vi "DMX.vi"(0 "Port Name":string, 1 "DMX channel no.":u8, 2 "Set value:":u8, 4 "Channel Name":string) -> (5 "Achieved value:":i32, 6 "error":bool)   [LabVIEW 2010]
panel:
  out "Read":string
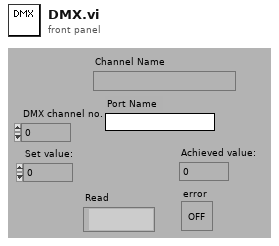
[diagram p1: front panel]
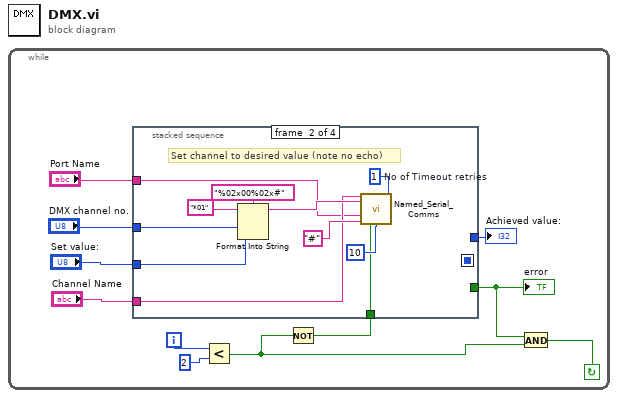
[diagram p0: block diagram]
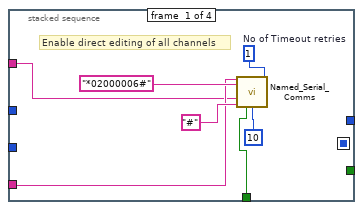
[diagram p2: hidden frame]
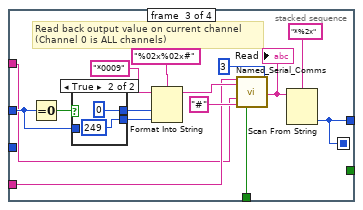
[diagram p3: hidden frame]
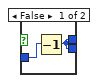
[diagram p4: hidden frame]
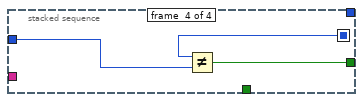
[diagram p5: hidden frame]
diagram:
  n1 = while {
    i -> [w7]
    stop <- w4 continue-if-true
    n2 = Less?(x=w7, y=2) -> (x < y?=w2:bool)
    n3 = Not(x=w2) -> (.not. x?=w1:bool)
    n4 = stacked-sequence {
      seq-local: [_ _ w34 _] -> [_ _ _ w51]
      tunnel: "DMX channel no." -> [_ w25 w37 _]
      tunnel: [_ _ w34 _] -> w10
      tunnel: [_ _ _ w50] -> w5
      tunnel: "Set value:" -> [_ w23 _ w49]
      tunnel: "Channel Name" -> [w15 w22 w33 _]
      tunnel: "Port Name" -> [w13 w20 w31 _]
      tunnel: w1 -> [w12 w19 w30 _]
      frame #0 {
        w14 = 1  # No of Timeout retries
        # "Enable direct editing of all channels"
        n5 = call "Named_Serial_Comms.vi"("Channel Name"=w15, "Write String"="*02000006#", "Timeout/ms"=u32 10, "!Timeout retries"=w14, "Port Name"=w13, "Term Grep"="#" ("Terminator"), "Log Errors?"=w12) -> ()  [unwired: 2 in, 7 out]
      }
      frame #1 {
        w21 = 1  # No of Timeout retries
        # "Set channel to desired value (note no echo)"
        n6 = Format Into String(format string="%02x00%02x#", initial string="*01", w25, w23) -> (resulting string=w27:string)  [unwired: 1 in, 1 out]
        n7 = call "Named_Serial_Comms.vi"("Channel Name"=w22, "Write String"=w27, "Timeout/ms"=u32 10, "!Timeout retries"=w21, "Port Name"=w20, "Term Grep"="#" ("Terminator"), "Log Errors?"=w19) -> ()  [unwired: 2 in, 7 out]
      }
      frame #2 {
        # "Read back output value on current channel\n(Channel 0 is ALL channels)"
        n8 = Equal To 0?(x=w37) -> (x = 0?=w38:bool)
        n9 = case shown="True" w38 {
          tunnel: w37 -> [w46 _]
          tunnel: [w45 u8 0 ("t")] -> w36
          tunnel: [w45 u8 249] -> w35
          frame False {
            n10 = Decrement(x=w46) -> (x-1=w45:u8)
          }
          frame True {
          }
        }
        n11 = Format Into String(format string="%02x%02x#", initial string="*0009", w36, w35) -> (resulting string=w42:string)  [unwired: 1 in, 1 out]
        n12 = call "Named_Serial_Comms.vi"("Channel Name"=w33, "Write String"=w42, "!Timeout retries"=3 ("No of Timeout retries"), "Port Name"=w31, "Term Grep"="#" ("Terminator"), "Log Errors?"=w30) -> ("Read"=w40:string)  [unwired: 3 in, 6 out]
        "Read" <- w40
        n13 = Scan From String(format string="*%2x", input string=w40) -> (output 1=w34:i32)  [unwired: 2 in, 4 out]
      }
      frame #3 {
        n14 = Not Equal?(x=w51, y=w49) -> (x != y?=w50:bool)
      }
    }
    "Achieved value:" <- w10
    "error" <- w5
    n15 = And(x=w5, y=w2) -> (x .and. y?=w4:bool)
  }
